vi "Write InstanceInfo.vi"(8 "error in (no error)":errorcluster, 10 "InstanceInfo":T1(array[cluster]), 11 "Polymorphic VI Type in":refnum<class "Polymorphic VI Type.lvclass">) -> (0 "error out":errorcluster, 3 "Polymorphic VI Type out":refnum<class "Polymorphic VI Type.lvclass">)   [LabVIEW 2020, in "Peek Window.lvlib" / "Polymorphic VI Type.lvclass"]
doc: "Basic write acceessor."
uses:
  Polymorphic VI Type.lvclass
  Polymorphic VI Type.lvclass/Polymorphic VI Type.ctl
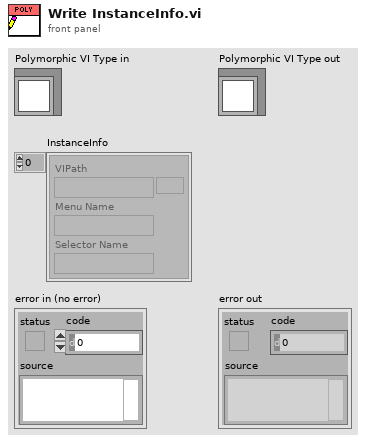
[diagram p1: front panel]
types:
  T1 = cluster{"VIPath":path, "Menu Name":string, "Selector Name":string}[]
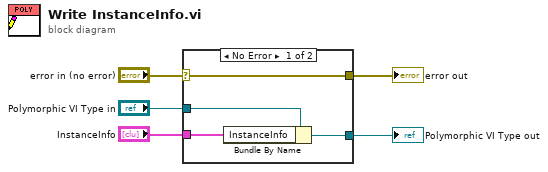
[diagram p0: block diagram]
diagram:
  n1 = case shown="No Error" "error in (no error)" {
    selector: "error in (no error)" -> [w9 w10]
    tunnel: [w9 w10] -> w4
    tunnel: [w7 w11] -> w2
    tunnel: "Polymorphic VI Type in" -> [w8 w11]
    tunnel: "InstanceInfo" -> [w6 _]
    frame No Error {
      n2 = Bundle By Name(cluster=w8, "InstanceInfo"=w6) -> (w7:refnum<class "Polymorphic VI Type.lvclass">)
    }
    frame Error {
    }
  }
  "error out" <- w4
  "Polymorphic VI Type out" <- w2
